vi "Write MsgPackMessage.vi"(8 "error in (no error)":errorcluster, 10 "wamplv.lvlib:MsgPackMessage.lvclass":refnum<class "MsgPackMessage.lvclass">, 11 "IMsgPackMessageHandler in":refnum<class "IMsgPackMessageHandler.lvclass">) -> (0 "error out":errorcluster, 3 "IMsgPackMessageHandler out":refnum<class "IMsgPackMessageHandler.lvclass">)   [LabVIEW 2020, in "wamplv.lvlib" / "IMsgPackMessageHandler.lvclass"]
uses:
  IMsgPackMessageHandler.lvclass
  IMsgPackMessageHandler.lvclass/IMsgPackMessageHandler.ctl
  SerialisedMessages/MsgPackMessage/MsgPackMessage.lvclass
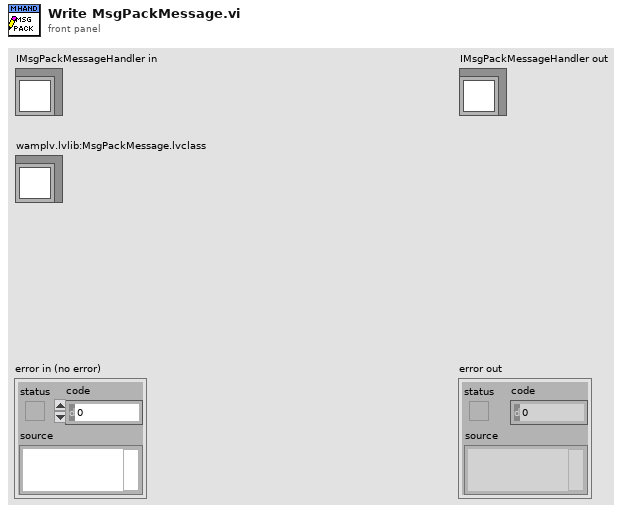
[diagram p1: front panel]
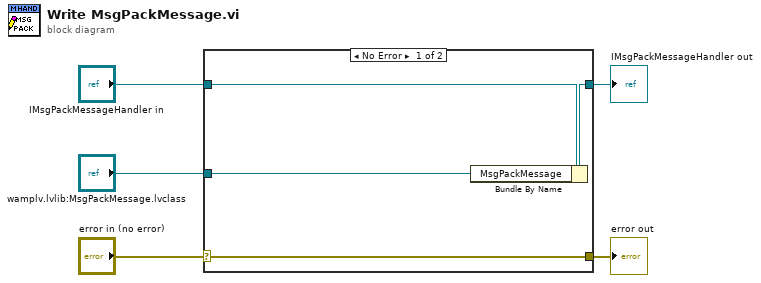
[diagram p0: block diagram]
diagram:
  n1 = case shown="No Error" "error in (no error)" {
    selector: "error in (no error)" -> [w9 w10]
    tunnel: [w9 w10] -> w4
    tunnel: [w7 w11] -> w2
    tunnel: "IMsgPackMessageHandler in" -> [w8 w11]
    tunnel: "wamplv.lvlib:MsgPackMessage.lvclass" -> [w6 _]
    frame No Error {
      n2 = Bundle By Name(cluster=w8, "MsgPackMessage"=w6) -> (w7:refnum<class "IMsgPackMessageHandler.lvclass">)
    }
    frame Error {
    }
  }
  "error out" <- w4
  "IMsgPackMessageHandler out" <- w2
